vi "Method.vi"(8 "error in":errorcluster, 9 "String":string, 10 "Numeric":dbl, 11 "Main in":refnum<class "Main.lvclass">) -> (0 "error out":errorcluster, 3 "Main out":refnum<class "Main.lvclass">)   [LabVIEW 2015, in "Main.lvlib" / "Main.lvclass"]
uses:
  Main.lvclass
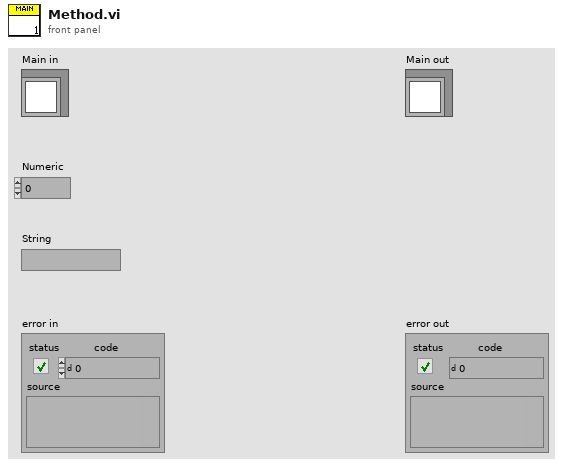
[diagram p1: front panel]
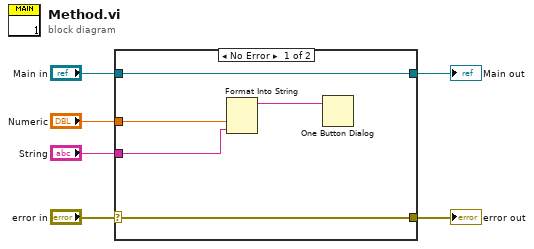
[diagram p0: block diagram]
diagram:
  n1 = case shown="No Error" "error in" {
    selector: "error in" -> [w10 w13]
    tunnel: [w10 w13] -> w5
    tunnel: [w11 w12] -> w3
    tunnel: "Main in" -> [w11 w12]
    tunnel: "Numeric" -> [w9 _]
    tunnel: "String" -> [w8 _]
    frame No Error {
      n2 = Format Into String(w9, w8) -> (resulting string=w7:string)  [unwired: 3 in, 1 out]
      n3 = One Button Dialog(message=w7) -> ()  [unwired: 1 in, 1 out]
    }
    frame Error {
    }
  }
  "error out" <- w5
  "Main out" <- w3
